vi "Status Registers.vi"(7 "Operation (F: Get)":bool, 8 "error in (no error)":errorcluster, 9 "Register (Status Byte)":i32(ring) items=["Status Byte (STB)", "Service Request Enable Register (SRE)", "Standard Event Status Register (ESR)", "Standard Event Status Enable Register (ESE)", "Error Status Register (ERRS)", "Error Status Enable Register (ERRE)", "Lock-In Status Register (LIAS)", "Lock-In Status Enable Register (LIAE)"], 10 "State (0)":u16, 11 "VISA Resource Name":refnum<visa-resource-name>) -> (0 "error out":errorcluster, 2 "State":u16, 3 "VISA Resource Name Out":refnum<visa-resource-name>)   [LabVIEW 2010, in "Stanford Research 844.lvlib"]
doc: "This Utility VI sets/gets the instrument status registers."
uses:
  <instrlib>/Stanford Research 844/Stanford Research 844.lvlib
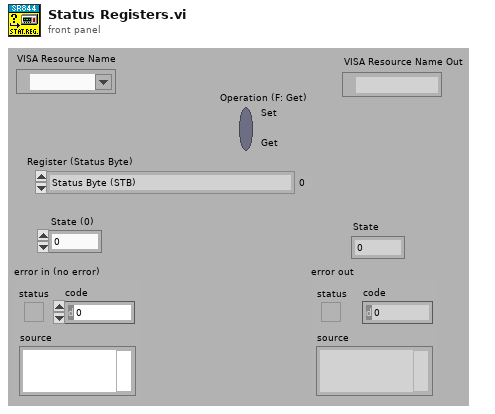
[diagram p1: front panel]
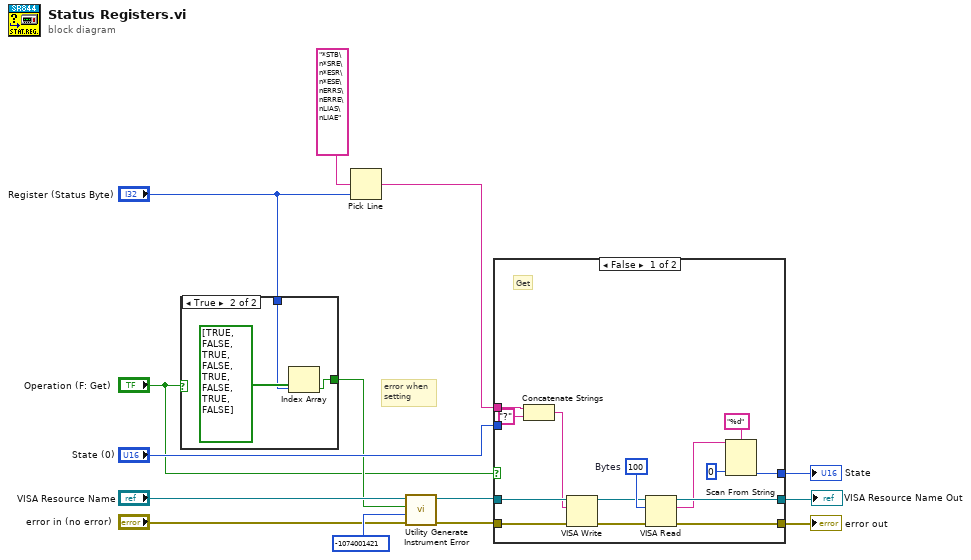
[diagram p0: block diagram]
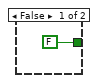
[diagram p2: hidden frame]
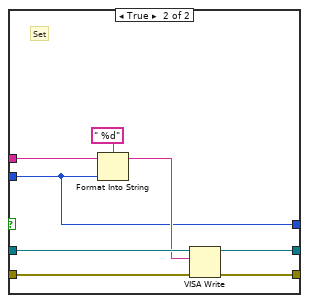
[diagram p3: hidden frame]
diagram:
  # "error when\nsetting"
  n1 = case shown="True" "Operation (F: Get)" {
    tunnel: "Register (Status Byte)" -> [_ w17]
    tunnel: [FALSE w16] -> w5
    frame False {
    }
    frame True {
      n2 = Index Array(array=bool[] [TRUE, FALSE, TRUE, FALSE, TRUE, FALSE, TRUE, FALSE] ("Array Constant"), index=w17) -> (element=w16:bool)
    }
  }
  n3 = Pick Line(multi-line string="*STB\n*SRE\n*ESR\n*ESE\nERRS\nERRE\nLIAS\nLIAE", line index="Register (Status Byte)") -> (output string=w12:string)  [unwired: 1 in]
  n4 = call <instrlib>:"Utility Generate Instrument Error.vi"("Error In"="error in (no error)", "Code (0)"=-1074001421 ("Error Code"), "Status (F: No error)"=w5, "VISA Resource Name"="VISA Resource Name") -> ("Error Out"=w2:errorcluster, "VISA Resource Name Out"=w6:refnum<visa-resource-name>)  [unwired: 6 in]
  n5 = case shown="False" "Operation (F: Get)" {
    tunnel: w6 -> [w27 w40]
    tunnel: w2 -> [w26 w39]
    tunnel: [w30 w38] -> w11
    tunnel: [w31 w37] -> w8
    tunnel: w12 -> [w20 w35]
    tunnel: "State (0)" -> [_ w33]
    tunnel: [w24 w33] -> w13
    frame False {
      w32 = u32 100  # Bytes
      # "Get"
      n6 = Concatenate Strings(w20, "?" ("string")) -> (w21:string)
      n7 = VISA Write(VISA resource name=w27, write buffer=w21, error in (no error)=w26) -> (VISA resource name out=w29:refnum<visa-resource-name>, error out=w28:errorcluster)  [unwired: 1 out]
      n8 = VISA Read(VISA resource name=w29, byte count=w32, error in (no error)=w28) -> (VISA resource name out=w31:refnum<visa-resource-name>, read buffer=w23:string, error out=w30:errorcluster)  [unwired: 1 out]
      n9 = Scan From String(format string="%d" ("Format String"), input string=w23, default 1=u16 0 ("Default Value 1")) -> (output 1=w24:u16)  [unwired: 2 in, 3 out]
    }
    frame True {
      # "Set"
      n10 = Format Into String(format string=" %d" ("Input Coupling"), initial string=w35, w33) -> (resulting string=w34:string)  [unwired: 1 in, 1 out]
      n11 = VISA Write(VISA resource name=w40, write buffer=w34, error in (no error)=w39) -> (VISA resource name out=w37:refnum<visa-resource-name>, error out=w38:errorcluster)  [unwired: 1 out]
    }
  }
  "error out" <- w11
  "State" <- w13
  "VISA Resource Name Out" <- w8
